vi "Data Type to Enum.vi"(7 "error in (no error)":errorcluster, 10 "datatype in":string) -> (0 "error out":errorcluster, 3 "UDV Data Type out":T1)   [LabVIEW 2016, in "Scan Engine Custom Device.lvlib"]
uses:
  Scan Engine Custom Device.lvlib
  Type Defs/UDV Data Type.ctl
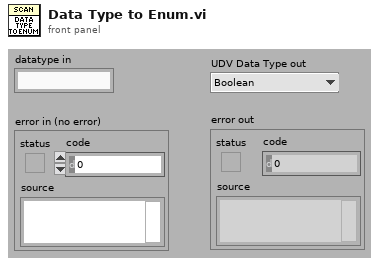
[diagram p1: front panel]
types:
  T1 = typedef "Scan Engine Custom Device.lvlib/UDV Data Type.ctl" = enum16{"Boolean", "Fixed Point", "Int8", "Int16", "Int32", "Int64", "U32 Bit Field", "UInt8", "UInt16", "UInt32", "UInt64", "Other"}
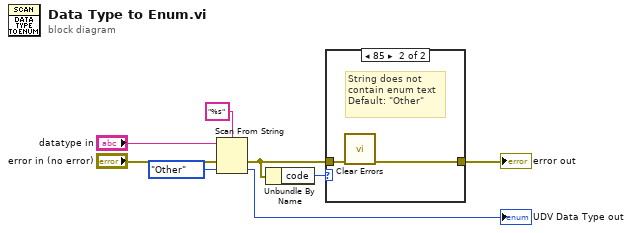
[diagram p0: block diagram]
diagram:
  n1 = Scan From String(format string="%s", input string="datatype in", error in="error in (no error)", default 1=UDV_Data_Type."Other" ("UDV Data Type")) -> (error out=w7:errorcluster, output 1=→"UDV Data Type out":T1)  [unwired: 1 in, 2 out]
  n2 = Unbundle By Name(w7) -> ("code"=w6:i32)
  n3 = case shown="85" w6 {
    tunnel: w7 -> [w9 w11]
    tunnel: [w9 w10] -> w1
    frame 0, Default {
    }
    frame 85 {
      # "String does not\ncontain enum text\nDefault: \"Other\""
      n4 = call <vilib>:"Clear Errors.vi"("error in (no error)"=w11) -> ("error out"=w10:errorcluster)  [unwired: 5 in, 1 out]
    }
  }
  "error out" <- w1
